vi "Gaussian.vi"(2 "Intput 3":u8[][](array[numeric]), 4 "seed":i32=-1, 5 "Input 2":u8[][](array[numeric]), 6 "standard deviation":dbl=1.0000000000000002 format="%0.2f", 7 "samples":i32, 8 "Amplify":dbl, 9 "right":i16, 10 "bottom":i16, 11 "Input 1":u8[][](array[numeric])) -> (0 "Output 3":u8[][](array[numeric]), 1 "Output 2":u8[][](array[numeric]), 3 "Output 1":u8[][](array[numeric]))   [LabVIEW 2016]
uses:
  <vilib>/Analysis/NI_AALBase.lvlib
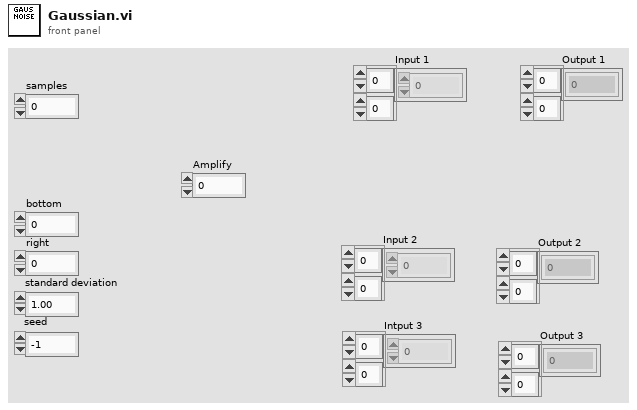
[diagram p1: front panel]
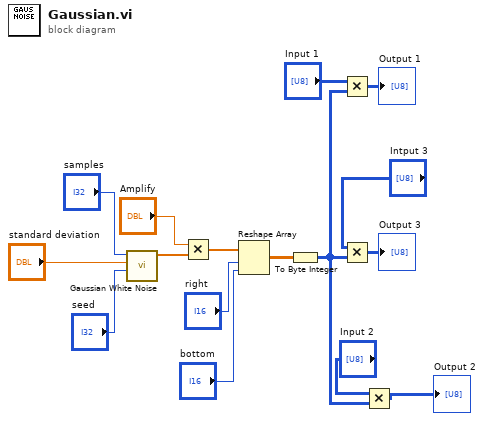
[diagram p0: block diagram]
diagram:
  n1 = call <vilib>:"Gaussian White Noise.vi"("seed"="seed", "standard deviation"="standard deviation", "samples"="samples") -> ("Gaussian noise pattern"=w12:dbl[])  [unwired: 7 in, 1 out]
  n2 = Multiply(x="Amplify", y=w12) -> (x*y=w13:dbl[])
  n3 = Reshape Array(w13, "right", "bottom") -> (w15:dbl[][])
  n4 = To Byte Integer(number=w15) -> (8bit integer=w1:i8[][])
  n5 = Multiply(x="Input 1", y=w1) -> (x*y=→"Output 1":u8[][])
  n6 = Multiply(x="Intput 3", y=w1) -> (x*y=→"Output 3":u8[][])
  n7 = Multiply(x="Input 2", y=w1) -> (x*y=→"Output 2":u8[][])
